vi "Co-Pilot Analyze.vi"(11 "JoystickDevRef":T1) -> (2 "Ejection":bool, 3 "Suction":bool, 4 "Fire Override":bool, 6 "Fire":bool)   [LabVIEW 2011]
uses:
  <vilib>/Rock Robotics/WPI/Joystick/WPI_JoystickDevRef.ctl
  <vilib>/Rock Robotics/WPI/Joystick/WPI_JoystickDeviceEnum.ctl
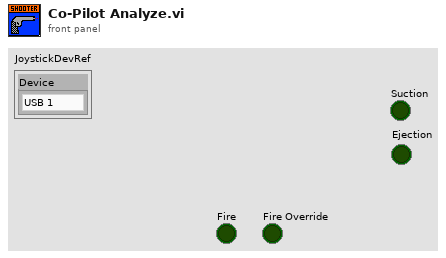
[diagram p1: front panel]
types:
  T1 = typedef "WPI_JoystickDevRef.ctl" = cluster{"Device":T2}
  T2 = typedef "WPI_JoystickDeviceEnum.ctl" = enum16{"USB 1", "USB 2", "USB 3", "USB 4", "Kinect 1", "Kinect 2"}
  T3 = typedef "WPI_JoystickButtonState.ctl" = cluster{"Button 1":bool, "Button 2":bool, "Button 3":bool, "Button 4":bool, "Button 5":bool, "Button 6":bool, "Button 7":bool, "Button 8":bool, "Button 9":bool, "Button 10":bool, "Button 11":bool, "Button 12":bool}
  T4 = cluster{"axis 1 (x)":dbl, "axis 2 (y)":dbl, "axis 3 (throttle)":dbl, "axis 4":dbl, "axis 5":dbl, "axis 6":dbl}
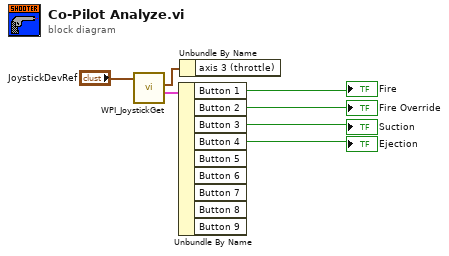
[diagram p0: block diagram]
diagram:
  n1 = call <vilib>:"WPI_JoystickGet.vi"("JoystickDevRef"="JoystickDevRef") -> ("Buttons"=w6:T3, "Axes"=w5:T4)  [unwired: 4 in, 1 out]
  n2 = Unbundle By Name(w6) -> ("Button 1"=→"Fire":bool, "Button 2"=→"Fire Override":bool, "Button 3"=→"Suction":bool, "Button 4"=→"Ejection":bool)  [unwired: 5 out]
  n3 = Unbundle By Name(w5) -> ()  [unwired: 1 out]
